vi "Make move.vi"(8 "error in (no error)":errorcluster, 10 "Move":refnum<class "Move.lvclass">, 11 "Position in":refnum<class "Position.lvclass">) -> (0 "error out":errorcluster, 3 "Position out":refnum<class "Position.lvclass">)   [LabVIEW 2015, in "Chesslib.lvlib" / "Position.lvclass"]
uses:
  Position.lvclass
  Moves/Move/Move.lvclass
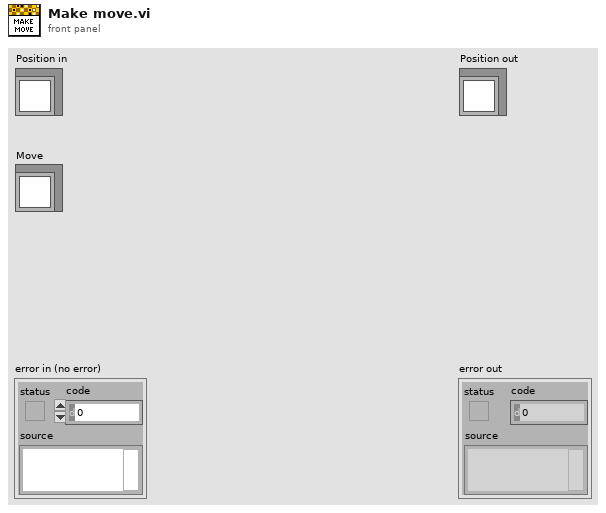
[diagram p1: front panel]
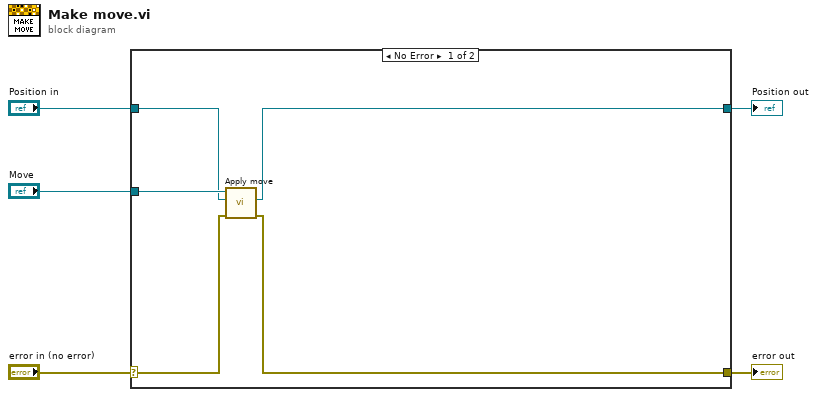
[diagram p0: block diagram]
diagram:
  n1 = case shown="No Error" "error in (no error)" {
    selector: "error in (no error)" -> [w8 w12]
    tunnel: [w7 w12] -> w4
    tunnel: [w6 w11] -> w2
    tunnel: "Position in" -> [w9 w11]
    tunnel: "Move" -> [w10 _]
    frame No Error {
      n2 = call "Apply move.vi"("error in (no error)"=w8, "Position in"=w9, "Move in"=w10) -> ("error out"=w7:errorcluster, "Position out"=w6:refnum<class "Position.lvclass">)  [unwired: 6 in, 1 out]
    }
    frame Error {
    }
  }
  "error out" <- w4
  "Position out" <- w2
